vi "HGF_SVEvent.appendData2Variant.vi"(2 "error in":errorcluster, 3 "SV Monitor Trigger":refnum<class "HGF_Event.lvclass">, 4 "initData":variant) -> (0 "error out":errorcluster, 1 "dup initData":variant)   [LabVIEW 2012, in "HGF_SV.lvlib" / "HGF_SVEvent.lvclass"]
uses:
  HGF_SVEvent.lvclass
  HGF_BaseClasses/HGF_Event/HGF_Event.lvclass
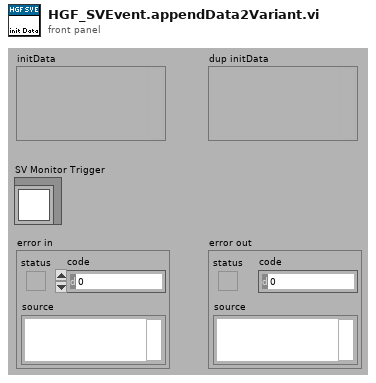
[diagram p1: front panel]
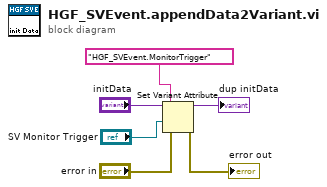
[diagram p0: block diagram]
diagram:
  n1 = Set Variant Attribute(Variant="initData", name="HGF_SVEvent.MonitorTrigger", value="SV Monitor Trigger", error in="error in") -> (Variant out=→"dup initData":variant, error out=→"error out":errorcluster)  [unwired: 1 out]
